vi "Operation Main.vi"(8 "error in (no error)":errorcluster, 11 "Front Panel Menu in":refnum<class "Front Panel Menu.lvclass">) -> (0 "error out":errorcluster, 3 "Front Panel Menu out":refnum<class "Front Panel Menu.lvclass">)   [LabVIEW 2024, in "Front Panel Menu.lvclass"]
uses:
  Front Panel Menu.lvclass
  Ancestor Class/Message/Message.lvclass/Message.ctl
  Ancestor Class/Message/Public Data/Read General CMD.vi
  Ancestor Class/Message/Public Data/Read CMD Type.vi
  Ancestor Class/Message/Message.lvclass
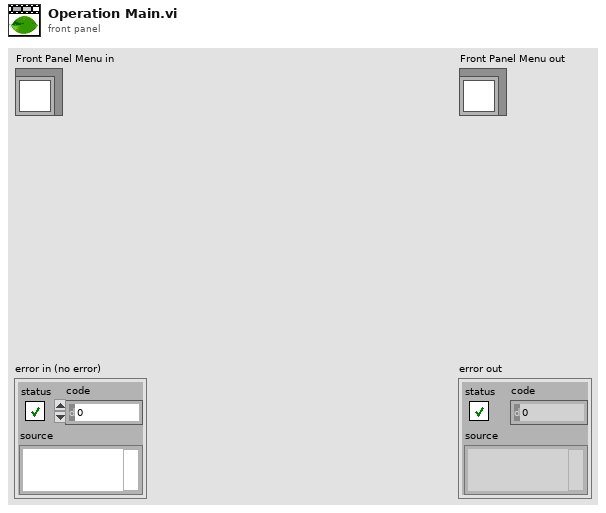
[diagram p1: front panel]
types:
  T1 = typedef "CMD Type.ctl" = enum16{"None", "General CMD", "1st CMD", "2nd CMD", "3rd CMD", "4th CMD", "5th CMD", "6th CMD", "7th CMD"}
  T2 = typedef "General CMD.ctl" = enum16{"None", "Stop", "Abort", "Running Task", "Running Batch Tasks", "Task Self Running", "Emergency Stop", "Subscribe", "UnSubscribe", "Pause", "Receive Parameters", "Active"}
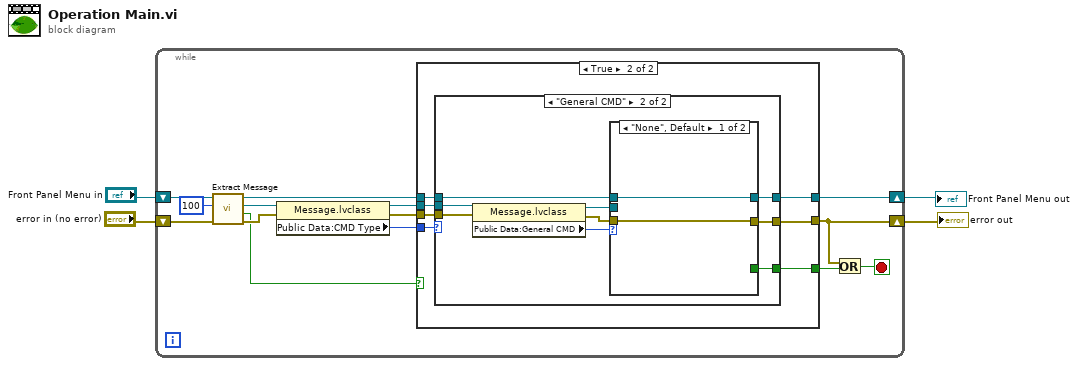
[diagram p0: block diagram]
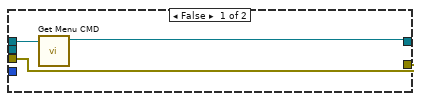
[diagram p2: hidden frame]
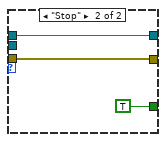
[diagram p4: hidden frame]
diagram:
  n1 = while {
    shift-right: [w9] -> w1
    shift-left: "Front Panel Menu in" -> [w14]
    shift-right: [w15] -> w3
    shift-left: "error in (no error)" -> [w13]
    stop <- w16 stop-if-true
    n2 = call-dynamic "Extract Message.vi"("error in (no error)"=w13, "Wait"=100, "System Actor in"=w14) -> ("error out"=w10:errorcluster, "Valid"=w5:bool, "Message Out"=w11:refnum<class "Message.lvclass">, "System Actor out"=w12:refnum<class "Front Panel Menu.lvclass">)  [unwired: 5 in]
    n3 = property class="Message.lvclass"(reference=w11, error in=w10) -> (reference out=w17:refnum<class "Message.lvclass">, error out=w7:errorcluster, "Public Data:CMD Type"=w18:T1)
    n4 = case shown="True" w5 {
      tunnel: w18 -> [_ w28]
      tunnel: w12 -> [w21 w26]
      tunnel: [w20 w25] -> w9
      tunnel: w17 -> [_ w27]
      tunnel: [w19 w24] -> w15
      tunnel: [_ w23] -> w8
      tunnel: w7 -> [w19 w22]
      frame False {
        n5 = call-dynamic "Get Menu CMD.vi"("Front Panel Menu in"=w21) -> ("Front Panel Menu out"=w20:refnum<class "Front Panel Menu.lvclass">)  [unwired: 8 in, 2 out]
      }
      frame True {
        n6 = case shown="\"General CMD\"" w28 {
          tunnel: w27 -> [_ w39]
          tunnel: w26 -> [w30 w36]
          tunnel: [w30 w33] -> w25
          tunnel: w22 -> [w29 w38]
          tunnel: [w29 w32] -> w24
          tunnel: [_ w31] -> w23
          frame "None", Default {
          }
          frame "General CMD" {
            n7 = property class="Message.lvclass"(reference=w39, error in=w38) -> (reference out=w35:refnum<class "Message.lvclass">, error out=w34:errorcluster, "Public Data:General CMD"=w37:T2)
            n8 = case shown="\"None\", Default" w37 {
              tunnel: w36 -> [w41 w44]
              tunnel: w35 -> [_ _]
              tunnel: w34 -> [w40 w43]
              tunnel: [w41 w44] -> w33
              tunnel: [w40 w43] -> w32
              tunnel: [_ TRUE] -> w31
              frame "None", Default {
              }
              frame "Stop" {
              }
            }
          }
        }
      }
    }
    n9 = Or(x=w15, y=w8) -> (x .or. y?=w16:bool)
  }
  "error out" <- w3
  "Front Panel Menu out" <- w1
